vi "Handshake.vi"(8 "error in (no error)":errorcluster, 11 "LocalQueueConnection in":refnum<class "LocalQueueConnection.lvclass">) -> (0 "error out":errorcluster, 3 "LocalQueueConnection out":refnum<class "LocalQueueConnection.lvclass">)   [LabVIEW 2013, in "MQTT_Queue.lvlib" / "LocalQueueConnection.lvclass"]
uses:
  LocalQueueConnection.lvclass
  MQTT_Connection/Connection/Connection.lvclass
  MQTT_Connection/Connection/Connection.lvclass/Connection.ctl
  LocalQueueConnection.lvclass/LocalQueueConnection.ctl
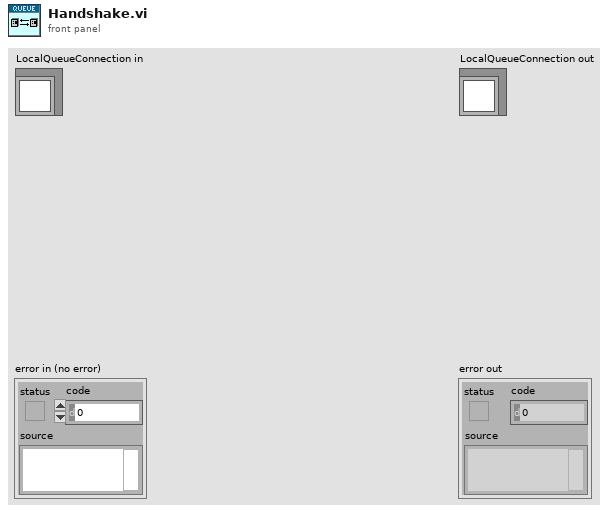
[diagram p1: front panel]
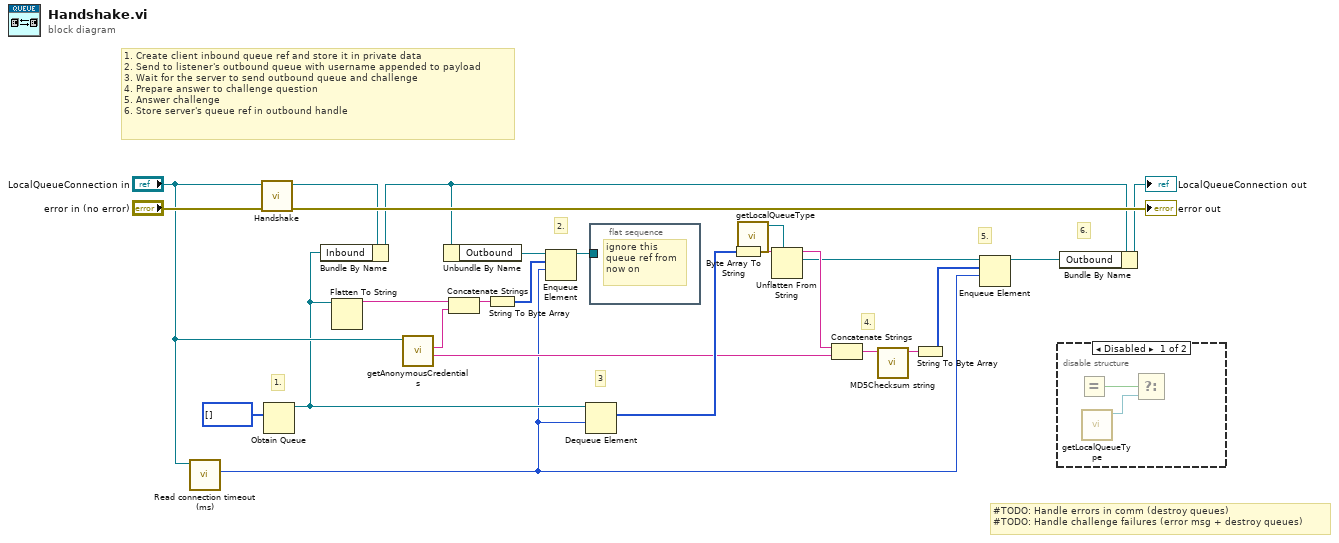
[diagram p0: block diagram]
diagram:
  # "6."
  # "5."
  # "4."
  # "#TODO: Handle errors in comm (destroy queues)\n#TODO: Handle challenge failures (error msg + destroy queues)"
  # "3"
  # "2."
  # "1. Create client inbound queue ref and store it in private data\n2. Send to listener's outbound queue with username appended to payload\n3. Wait for the server to send outbound queue and challenge\n4. Prepare answer to challenge question\n5. Answer challenge\n6. Store server's queue ref in outbound handle"
  # "1."
  n1 = call "Read connection timeout (ms).vi"("Connection in"="LocalQueueConnection in") -> ("connection timeout (ms)"=w1:i32)  [unwired: 8 in, 2 out]
  n2 = call-parent "Handshake.vi"("error in (no error)"="error in (no error)", "Connection in"="LocalQueueConnection in") -> ("error out"=→"error out":errorcluster, "Connection out"=w15:refnum<class "LocalQueueConnection.lvclass">)  [unwired: 8 in]
  n3 = Obtain Queue(element data type=u8[] [] ("Bytes")) -> (queue out=w13:refnum<queue>)  [unwired: 4 in, 2 out]
  n4 = Bundle By Name(cluster=w15, "Inbound"=w13) -> (w12:refnum<class "LocalQueueConnection.lvclass">)
  n5 = Flatten To String(anything=w13) -> (data string=w19:string)  [unwired: 3 in, 2 out]
  n6 = call "getAnonymousCredentials.vi"("LocalQueueConnection"="LocalQueueConnection in") -> ("Anonymous password"=w7:string, "Anonymous username"=w20:string)  [unwired: 9 in]
  n7 = Unbundle By Name(w12) -> ("Outbound"=w22:refnum<queue>)
  n8 = Concatenate Strings(w19, w20) -> (w18:string)
  n9 = String To Byte Array(string=w18) -> (unsigned byte array=w21:u8[])
  n10 = Enqueue Element(queue=w22, element=w21, timeout in ms (-1)=w1) -> (queue out=w16:refnum<queue>)  [unwired: 1 in, 2 out]
  n11 = Dequeue Element(queue=w13, timeout in ms (-1)=w1) -> (element=w8:u8[])  [unwired: 1 in, 3 out]
  n12 = flat-sequence {
    tunnel: w16 -> [_]
    frame #0 {
      # "ignore this\nqueue ref from\nnow on"
    }
  }
  n13 = Byte Array To String(unsigned byte array=w8) -> (string=w9:string)
  n14 = call "getLocalQueueType.vi"() -> ("Queue Type"=w10:refnum<queue>)  [unwired: 11 in]
  n15 = Unflatten From String(type=w10, binary string=w9) -> (rest of the binary string=w6:string, value=w5:refnum<queue>)  [unwired: 3 in, 1 out]
  n16 = Concatenate Strings(w6, w7) -> (w17:string)
  n17 = call <vilib>:"MD5Checksum string.vi"("Message String"=w17) -> ("MD5 message-digest"=w3:string)  [unwired: 10 in]
  n18 = String To Byte Array(string=w3) -> (unsigned byte array=w2:u8[])
  n19 = Enqueue Element(queue=w5, element=w2, timeout in ms (-1)=w1) -> (queue out=w4:refnum<queue>)  [unwired: 1 in, 2 out]
  n20 = disable-structure shown="Disabled" {
    frame Disabled {
      n21 = Equal?() -> (x = y?=w27:bool)  [unwired: 2 in]
      n22 = call "getLocalQueueType.vi"() -> ("Queue Type"=w26:refnum<queue>)  [unwired: 11 in]
      n23 = Select(s=w27, f=w26) -> ()  [unwired: 1 in, 1 out]
    }
    frame Enabled {
    }
  }
  n24 = Bundle By Name(cluster=w12, "Outbound"=w4) -> (→"LocalQueueConnection out":refnum<class "LocalQueueConnection.lvclass">)
